vi "Link Channel Core.vi"(8 "error in (no error)":errorcluster, 10 "Channel Connection":T1, 11 "CIF_UI in":refnum<class "CIF_UI.lvclass">) -> (0 "error out":errorcluster, 3 "CIF_UI out":refnum<class "CIF_UI.lvclass">)   [LabVIEW 2021, in "CIF_UI.lvclass"]
uses:
  CIF_UI.lvclass
  Typedef/Channel Connection.ctl
  CIF_UI.lvclass/CIF_UI.ctl
  CIFCore/Grpc/CIFCoreChannel_client/RPC Messages/cif_channelcore_ConnectSubscriber.ctl
  CIFCore/Common/Typedef/Errors.ctl
  CIFCore/Common/Utilities/Append Error Location.vi
  CIFCore/Grpc/CIFCoreWrapper/CIFCoreWrapper.lvlib
  CIFCore/Grpc/CIFCoreChannel_client/CIFCoreChannel_client.lvlib
  CIFCore/Common/CIFCoreCommon.lvlib
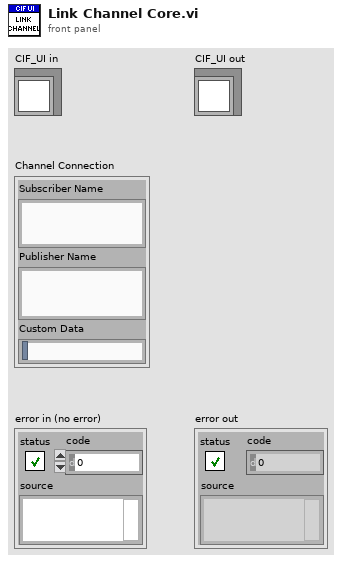
[diagram p1: front panel]
types:
  T1 = typedef "CIF_UI.lvclass/Channel Connection.ctl" = cluster{"Subscriber Name":string, "Publisher Name":string, "Custom Data":string}
  T2 = typedef "CIF_UI.lvclass/Plugin Connection Map.ctl" = map{string, T3}
  T3 = typedef "CIF_UI.lvclass/Plugin Connections.ctl" = cluster{"gRPC ID":T4, "Plugin info":T5}
  T4 = typedef "grpc-lvsupport-release.lvlib/grpcId.ctl" = u64
  T5 = typedef "CIF_Manager_client.lvlib/cif_manager_PluginInfo.ctl" = cluster{"plugin_name":string, "plugin_type":string, "grpc_port":i32, "plugin_version":T6, "status":T7}
  T6 = typedef "CIF_Manager_client.lvlib/cif_manager_PluginVersion.ctl" = cluster{"major_version":i32, "minor_version":i32, "fix_version":i32, "build_version":i32}
  T7 = typedef "CIF_Manager_client.lvlib/cif_plugincore_StatusData.ctl" = cluster{"state":T8, "timing_statistics":T9, "fifo_statistics":T11, "error":T12, "monitor_doubles":T13, "monitor_u64s":T14, "monitor_i64s":T15}
  T8 = typedef "CIF_Manager_client.lvlib/cif_plugincore_StatusData_State.ctl" = enum32{"NULL", "CREATING", "LISTENING", "RUNNING", "CLEANINGUP", "DESTROYING"}
  T9 = typedef "CIF_Manager_client.lvlib/cif_plugincore_TimingStatistics.ctl" = cluster{"period":T10, "wake_error":T10, "execute":T10, "housekeep":T10, "idle":T10}
  T10 = typedef "CIF_Manager_client.lvlib/cif_plugincore_TimingStatsBasic.ctl" = cluster{"max":i32, "min":i32}
  T11 = typedef "CIF_Manager_client.lvlib/cif_plugincore_FifoStatistics.ctl" = cluster{"from_t0":T10, "from_previous_plugin":T10, "output_error":T10}
  T12 = typedef "CIF_Manager_client.lvlib/cif_plugincore_Error.ctl" = cluster{"status":bool, "code":i32}
  T13 = typedef "CIF_Manager_client.lvlib/cif_plugincore_MonitorDoubles.ctl" = cluster{"double_1":dbl, "double_2":dbl, "double_3":dbl, "double_4":dbl}
  T14 = typedef "CIF_Manager_client.lvlib/cif_plugincore_MonitorU64.ctl" = cluster{"u64_1":u64, "u64_2":u64, "u64_3":u64, "u64_4":u64}
  T15 = typedef "CIF_Manager_client.lvlib/cif_plugincore_MonitorI64.ctl" = cluster{"i64_1":i64, "i64_2":i64, "i64_3":i64, "i64_4":i64}
  T16 = typedef "CIFCoreChannel_client.lvlib/cif_channelcore_ConnectSubscriber.ctl" = cluster{"subscriber_name":string, "publisher_name":string, "custom_connect":u8[]}
  T17 = typedef "CIFCoreCommon.lvlib/Errors.ctl" = enum16{"Invalid Clock ID", "Long Sleep", "gRPC Server Not Found", "Config Parse", "Timestamp Wrap", "Delayed Execution", "Duplicate Channel", "Missing Channel", "Incorrect Type", "Flatten Error", "Unflatten Data", "Unique Name", "Plugin Not Found", "Plugin Type Not Found", "Plugin Version Not Found", "Manager Not Found", "Numerical Issue", "Time Jump", "Clock ID Match", "Channel Length", "Plugin Connection", "gRPC Server Connection"}
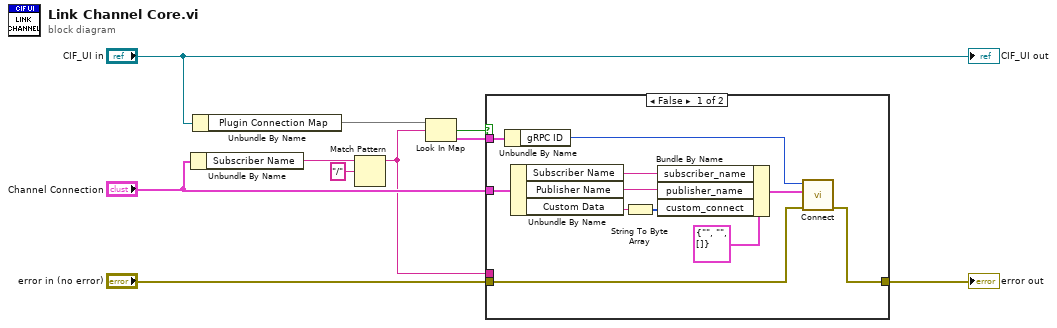
[diagram p0: block diagram]
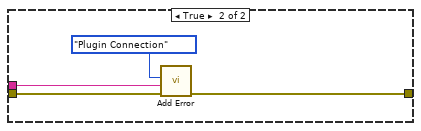
[diagram p2: hidden frame]
diagram:
  n1 = Unbundle By Name("Channel Connection") -> ("Subscriber Name"=w6:string)
  n2 = Unbundle By Name("CIF_UI in") -> ("Plugin Connection Map"=w9:T2)
  n3 = Match Pattern(string=w6, regular expression="/") -> (before substring=w2:string)  [unwired: 1 in, 3 out]
  n4 = Look In Map(map=w9, key=w2) -> (key not found?=w4:bool, value=w3:T3)  [unwired: 1 in]
  n5 = case shown="False" w4 {
    tunnel: "error in (no error)" -> [w12 w25]
    tunnel: w3 -> [w21 _]
    tunnel: "Channel Connection" -> [w13 _]
    tunnel: [w11 w24] -> w8
    tunnel: w2 -> [_ w23]
    frame False {
      n6 = Unbundle By Name(w21) -> ("gRPC ID"=w14:T4)
      n7 = Unbundle By Name(w13) -> ("Subscriber Name"=w20:string, "Publisher Name"=w19:string, "Custom Data"=w17:string)
      n8 = String To Byte Array(string=w17) -> (unsigned byte array=w18:u8[])
      n9 = Bundle By Name(cluster=T16 {"subscriber_name"="", "publisher_name"="", "custom_connect"=[]} ("Connection 2"), "subscriber_name"=w20, "publisher_name"=w19, "custom_connect"=w18) -> (w15:T16)
      n10 = call "Connect.vi"("error in"=w12, "Connection"=w15, "gRPC ID"=w14) -> ("error out"=w11:errorcluster)  [unwired: 7 in, 1 out]
    }
    frame True {
      n11 = call "Add Error.vi"("error in (no error)"=w25, "String to Append"=w23, "Error"=Errors."Plugin Connection") -> ("error out"=w24:errorcluster)  [unwired: 8 in]
    }
  }
  "error out" <- w8
  "CIF_UI out" <- "CIF_UI in"
